vi "Teleop - shooter shoot (SubVI).vi"(0 "Boolean":bool, 1 "33. shooterSerializerSpeed in":dbl, 2 "shooterAngleDesired":dbl, 3 "serializerOutput":dbl, 4 "offsetAngle H":dbl, 6 "shooterVelocity":dbl, 7 "32. shooterAngleRange":dbl, 8 "shooterAnglePosition":dbl, 9 "31. turretHRange":dbl, 10 "targetLock?":bool, 11 "29. shooterVelocityUpperLimit":dbl, 13 "30. shooterVelocityLowerLimit":dbl) -> (14 "33. shooterSerializerSpeed out":dbl)   [LabVIEW 2019]
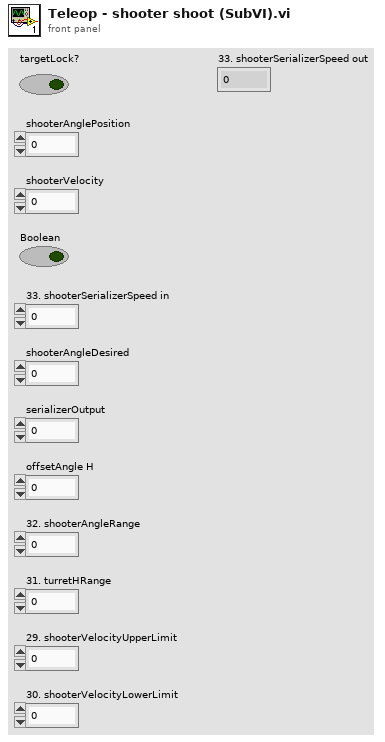
[diagram p1: front panel]
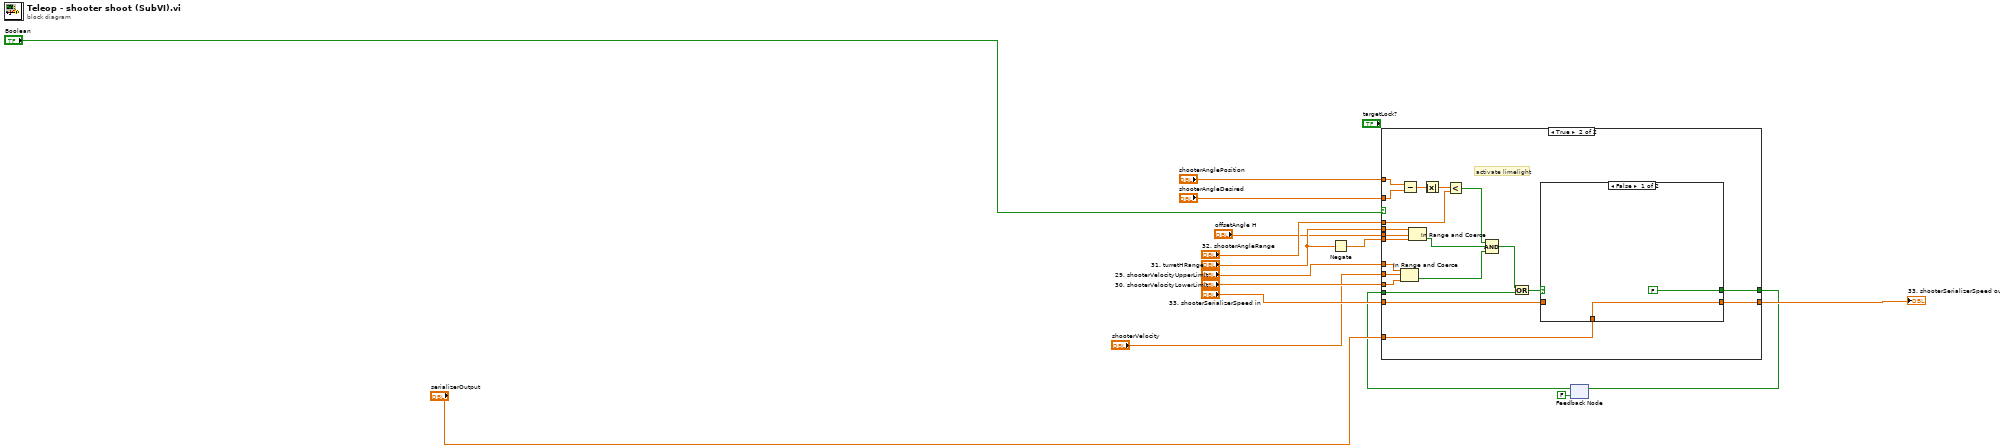
[diagram p0: block diagram]
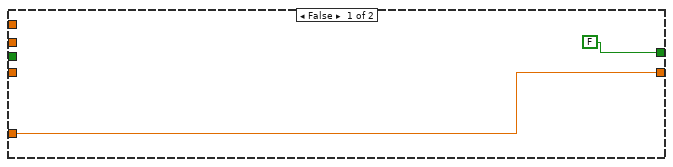
[diagram p2: hidden frame]
diagram:
  n1 = Negate(x="31. turretHRange") -> (-x=w10:dbl)
  n2 = feedback #1(FALSE) -> (w6:bool)
  n3 = case shown="True" "Boolean" {
    tunnel: "shooterVelocity" -> [_ w39]
    tunnel: "29. shooterVelocityUpperLimit" -> [_ w38]
    tunnel: "30. shooterVelocityLowerLimit" -> [_ w37]
    tunnel: [FALSE w36] -> w5
    tunnel: w6 -> [_ w35]
    tunnel: "offsetAngle H" -> [_ w33]
    tunnel: "31. turretHRange" -> [_ w32]
    tunnel: w10 -> [_ w31]
    tunnel: "shooterAngleDesired" -> [_ w29]
    tunnel: "shooterAnglePosition" -> [_ w30]
    tunnel: "32. shooterAngleRange" -> [_ w27]
    tunnel: [w17 w21] -> w14
    tunnel: "33. shooterSerializerSpeed in" -> [_ w20]
    tunnel: "serializerOutput" -> [w17 w19]
    frame False {
    }
    frame True {
      # "activate limelight"
      n4 = In Range and Coerce(upper limit=w38, x=w39, lower limit=w37) -> (In Range?=w22:bool)  [unwired: 1 out]
      n5 = Subtract(x=w30, y=w29) -> (x-y=w28:dbl)
      n6 = In Range and Coerce(upper limit=w32, x=w33, lower limit=w31) -> (In Range?=w23:bool)  [unwired: 1 out]
      n7 = Absolute Value(x=w28) -> (abs(x)=w26:dbl)
      n8 = Less?(x=w26, y=w27) -> (x < y?=w24:bool)
      n9 = Compound Arithmetic op=AND(w24, w23, w22) -> (w25:bool)
      n10 = Or(x=w25, y=w35) -> (x .or. y?=w34:bool)
      n11 = case shown="False" w34 {
        selector: w34 -> [_ w43]
        tunnel: [FALSE w43] -> w36
        tunnel: [w40 w42] -> w21
        tunnel: w20 -> [_ w42]
        tunnel: w19 -> [w40 _]
        frame False {
        }
        frame True {
        }
      }
    }
  }
  "33. shooterSerializerSpeed out" <- w14
  n12 = feedback-in #1(w5) -> ()
